vi "saveEvent.vi"(8 "error in (no error)":errorcluster, 11 "WinX32Settings in":refnum<class "WinX32Settings.lvclass">) -> (0 "error out":errorcluster, 3 "WinX32Settings out":refnum<class "WinX32Settings.lvclass">)   [LabVIEW 2011, in "Tools.lvlib" / "Settings.lvlib" / "WinX32Settings.lvclass"]
uses:
  WinX32Settings.lvclass
  WinX32Settings.lvclass/WinX32Settings.ctl
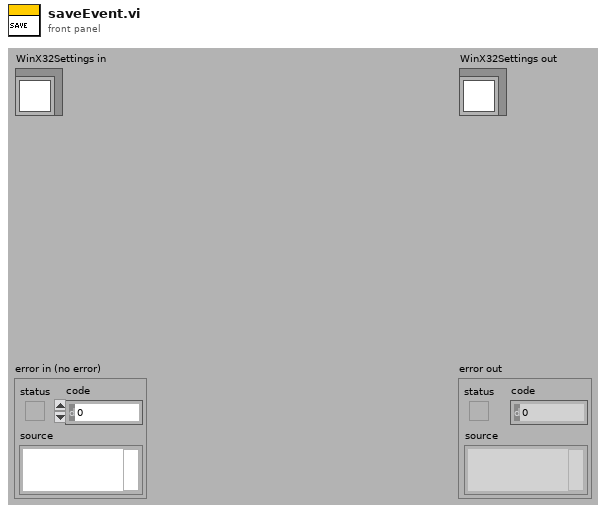
[diagram p1: front panel]
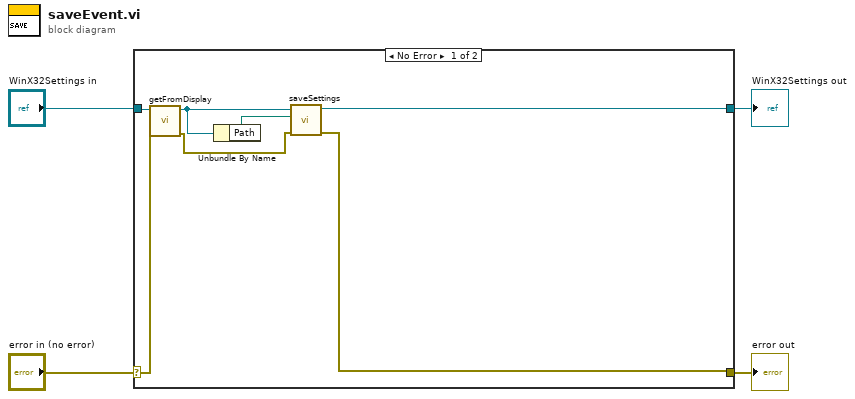
[diagram p0: block diagram]
diagram:
  n1 = case shown="No Error" "error in (no error)" {
    selector: "error in (no error)" -> [w6 w13]
    tunnel: [w10 w13] -> w3
    tunnel: [w9 w12] -> w1
    tunnel: "WinX32Settings in" -> [w8 w12]
    frame No Error {
      n2 = call "getFromDisplay.vi"("error in (no error)"=w6, "WinX32Settings in"=w8) -> ("error out"=w5:errorcluster, "WinX32Settings out"=w7:refnum<class "WinX32Settings.lvclass">)  [unwired: 8 in]
      n3 = Unbundle By Name(w7) -> ("Path"=w11:path)
      n4 = call-dynamic "saveSettings.vi"("error in (no error)"=w5, "Path"=w11, "WinX32Settings in"=w7) -> ("error out"=w10:errorcluster, "WinX32Settings out"=w9:refnum<class "WinX32Settings.lvclass">)  [unwired: 7 in]
    }
    frame Error {
    }
  }
  "error out" <- w3
  "WinX32Settings out" <- w1
